vi "Messenger Initialize.vi"(7 "Elements Of Container":i32=1, 8 "error in (no error)":errorcluster, 9 "Paras In 2":variant, 10 "Paras In":variant, 11 "Simple Map Queue Group Messenger in":refnum<class "Simple Map Queue Group Messenger.lvclass">) -> (0 "error out":errorcluster, 3 "Simple Map Queue Group Messenger out":refnum<class "Simple Map Queue Group Messenger.lvclass">)   [LabVIEW 2024, in "Simple Map Queue Group Messenger.lvclass"]
uses:
  Simple Map Queue Group Messenger.lvclass
  TypeDef/Queue Group Map.ctl
  Simple Tree Queue Messenger/Type Def/Message Queue.ctl
  Ancestor Class/Message/Message.lvclass
  Simple Map Queue Group Messenger.lvclass/Simple Map Queue Group Messenger.ctl
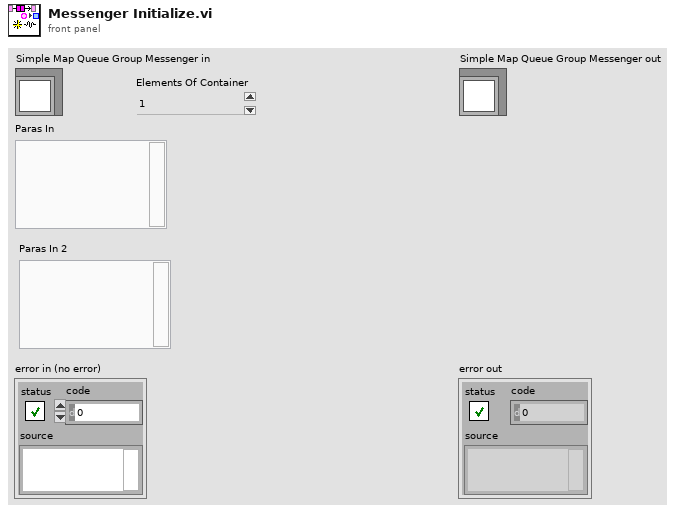
[diagram p1: front panel]
types:
  T1 = typedef "Queue Group Map.ctl" = map{i64, T2[]}
  T2 = typedef "Message Queue.ctl" = refnum<queue>
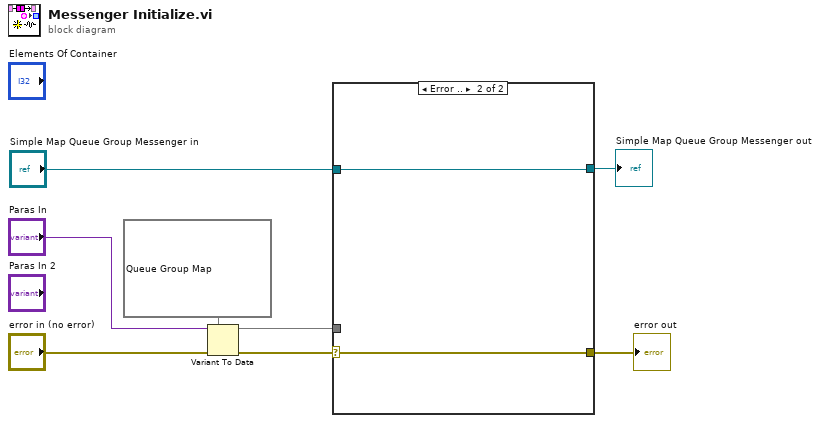
[diagram p0: block diagram]
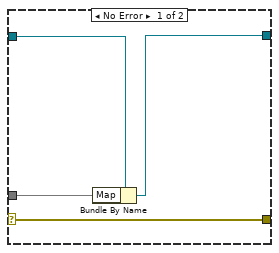
[diagram p2: hidden frame]
diagram:
  n1 = Variant To Data(error in="error in (no error)", type=T1 {} ("Map"), Variant="Paras In") -> (data=w4:T1, error out=w5:errorcluster)
  n2 = case shown="Error .." w5 {
    selector: w5 -> [w12 w13]
    tunnel: w4 -> [w10 _]
    tunnel: "Simple Map Queue Group Messenger in" -> [w11 w14]
    tunnel: [w12 w13] -> w2
    tunnel: [w9 w14] -> w1
    frame No Error {
      n3 = Bundle By Name(cluster=w11, "Map"=w10) -> (w9:refnum<class "Simple Map Queue Group Messenger.lvclass">)
    }
    frame Error {
    }
  }
  "error out" <- w2
  "Simple Map Queue Group Messenger out" <- w1
